vi "Single Float Value.vi"(8 "error in (no error)":errorcluster, 11 "Double Float in":refnum<class "Complex Extended Float.lvclass">) -> (0 "error out":errorcluster, 2 "Float":sgl, 3 "Double Float out":refnum<class "Complex Extended Float.lvclass">)   [LabVIEW 2021, in "Complex Extended Float.lvclass"]
uses:
  Complex Extended Float.lvclass
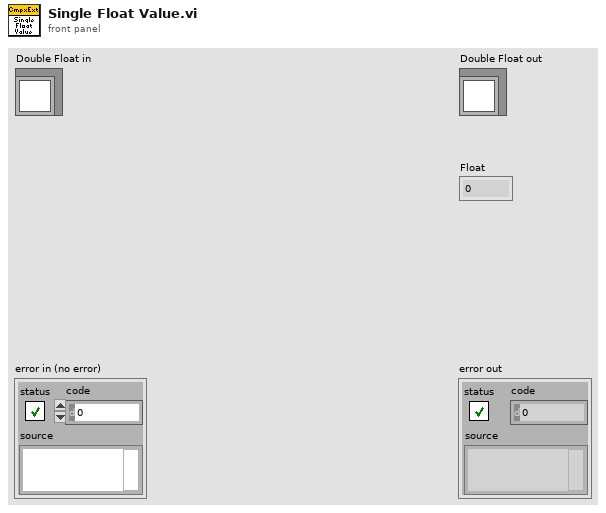
[diagram p1: front panel]
types:
  T1 = typedef "Complex Extended Float.lvclass/Type.ctl" = cxt
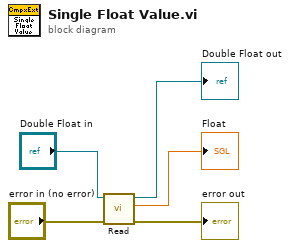
[diagram p0: block diagram]
diagram:
  n1 = call-dynamic "Read.vi"("error in (no error)"="error in (no error)", "Double Float.lvclass_340760 in"="Double Float in") -> ("error out"=→"error out":errorcluster, "Value"=→"Float":T1, "Double Float.lvclass_340760 out"=→"Double Float out":refnum<class "Complex Extended Float.lvclass">)  [unwired: 7 in]
